vi "Close Shutters.vi"(8 "error in (no error)":errorcluster) -> (0 "error out (no error)":errorcluster)   [LabVIEW 2017]
uses:
  Typedefs/PMT control functions.ctl
  Typedefs/Shutter Function Enum.ctl
  Global Variables/General Globals.vi
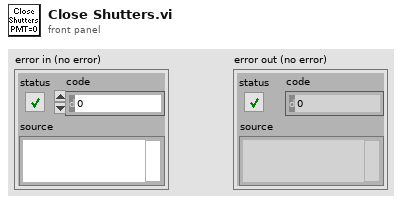
[diagram p1: front panel]
types:
  T1 = typedef "Shutter Function Enum.ctl" = enum16{"Open Shutter", "Close Shutter"}
  T2 = typedef "PMT control functions.ctl" = enum16{"Set PMTs from UI", "Reset PMTs"}
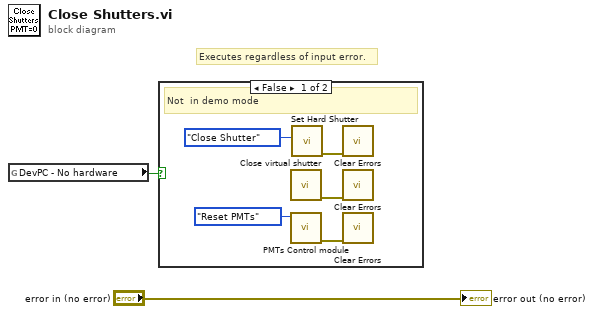
[diagram p0: block diagram]
diagram:
  # "Executes regardless of input error."
  n1 = global read "General Globals.vi" "DevPC - No hardware"() -> (w1:bool)
  n2 = case shown="False" w1 {
    frame False {
      # "Not  in demo mode"
      n3 = call "Close virtual shutter.vi"() -> ("error out"=w5:errorcluster)  [unwired: 11 in]
      n4 = call "PMTs Control module.vi"("Function"=PMT_control_functions."Reset PMTs") -> ("Error Out"=w6:errorcluster)  [unwired: 10 in]
      n5 = call "Set Hard Shutter.vi"("Shutter Function"=Shutter_Function_Enum."Close Shutter") -> ("Error Out"=w3:errorcluster)  [unwired: 10 in]
      n6 = call <vilib>:"Clear Errors.vi"("error in (no error)"=w3) -> ()  [unwired: 5 in, 2 out]
      n7 = call <vilib>:"Clear Errors.vi"("error in (no error)"=w5) -> ()  [unwired: 5 in, 2 out]
      n8 = call <vilib>:"Clear Errors.vi"("error in (no error)"=w6) -> ()  [unwired: 5 in, 2 out]
    }
    frame True {
      # "Demo mode"
    }
  }
  "error out (no error)" <- "error in (no error)"
